vi "Get Angles.vi"(11 "Array in":refnum<vi>) -> (2 "Relative Change":dbl[](array[numeric]), 3 "Angles":dbl[](array[numeric]))   [LabVIEW 2025]
panel:
  out "element":i32
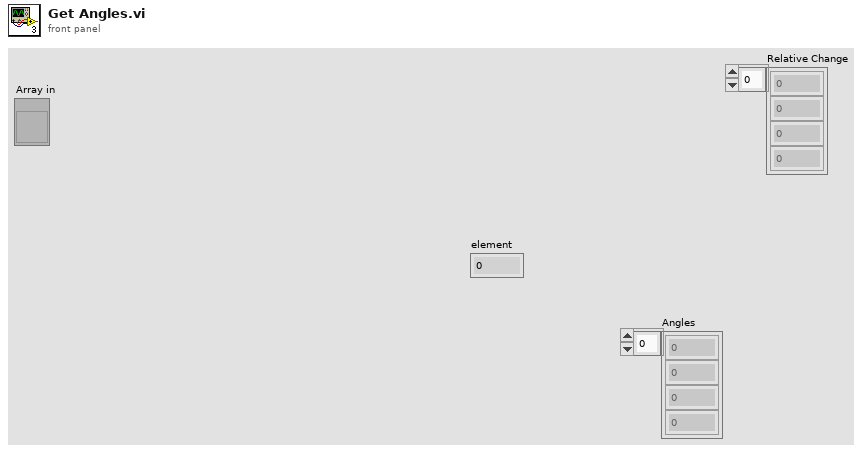
[diagram p1: front panel]
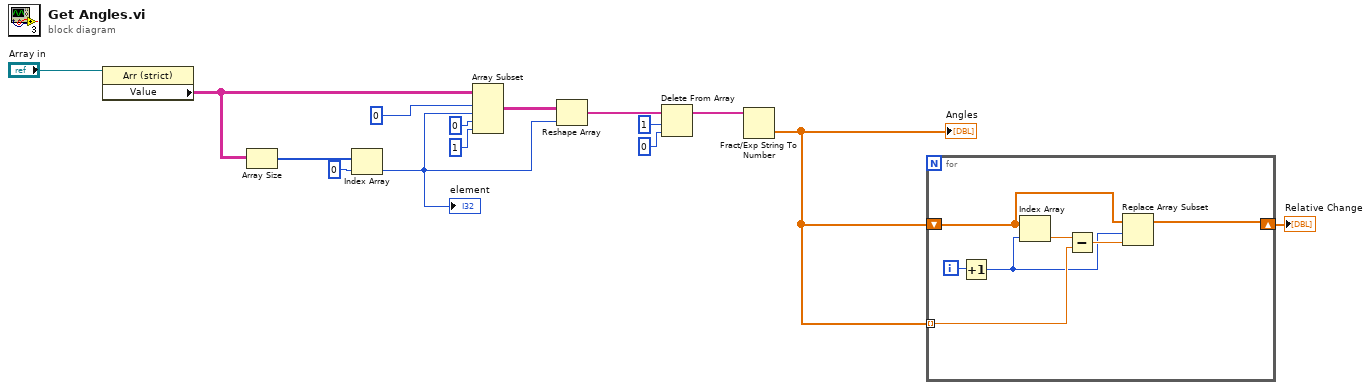
[diagram p0: block diagram]
diagram:
  n1 = property class="Arr (strict)"(reference="Array in") -> ("Value"=w12:string[][])  [unwired: 1 in, 2 out]
  n2 = Array Size(array=w12) -> (size(s)=w14:i32[])
  n3 = Index Array(array=w14, index=0) -> (element=w7:i32)
  "element" <- w7
  n4 = Array Subset(array=w12, index (row)=0 ("index"), length (row)=w7, index (col)=0 ("index"), length (col)=1 ("length")) -> (w8:string[][])
  n5 = Reshape Array(w8, w7) -> (w6:string[])
  n6 = Delete From Array(array=w6, length=1, index=0) -> (array with subset deleted=w3:string[])  [unwired: 1 out]
  n7 = Fract/Exp String To Number(string=w3) -> (number=w2:dbl[])  [unwired: 3 in, 1 out]
  "Angles" <- w2
  n8 = for {
    tunnel: w2 -> [w20] mode=indexing
    shift-right: [w16] -> w1
    shift-left: w2 -> [w19]
    i -> [w22]
    n9 = Increment(x=w22) -> (x+1=w17:i32)
    n10 = Index Array(array=w19, index=w17) -> (element=w21:dbl)
    n11 = Subtract(x=w21, y=w20) -> (x-y=w18:dbl)
    n12 = Replace Array Subset(array=w19, new element=w18, index=w17) -> (w16:dbl[])
  }
  "Relative Change" <- w1
